vi "MeasureAndSaveData.vi"(0 "object in":refnum<class "AD2_SDK.lvclass">, 2 "tdms file":refnum<k34>, 5 "error in (no error)":errorcluster) -> (14 "object out":refnum<class "AD2_SDK.lvclass">, 17 "Channels array":waveform(dbl)[](array[waveform]), 19 "error out":errorcluster)   [LabVIEW 2023, in "AD2_SDK.lvclass"]
uses:
  AD2_SDK.lvclass
  AD2_SDK.lvclass/AD2_SDK.ctl
  <vilib>/measure/NI_MAPro.lvlib
  <vilib>/measure/matone.llb/Extract Single Tone Information 1 Chan.vi
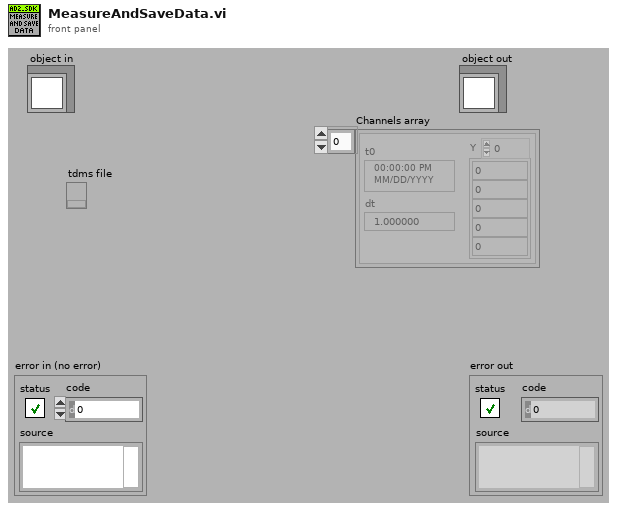
[diagram p1: front panel]
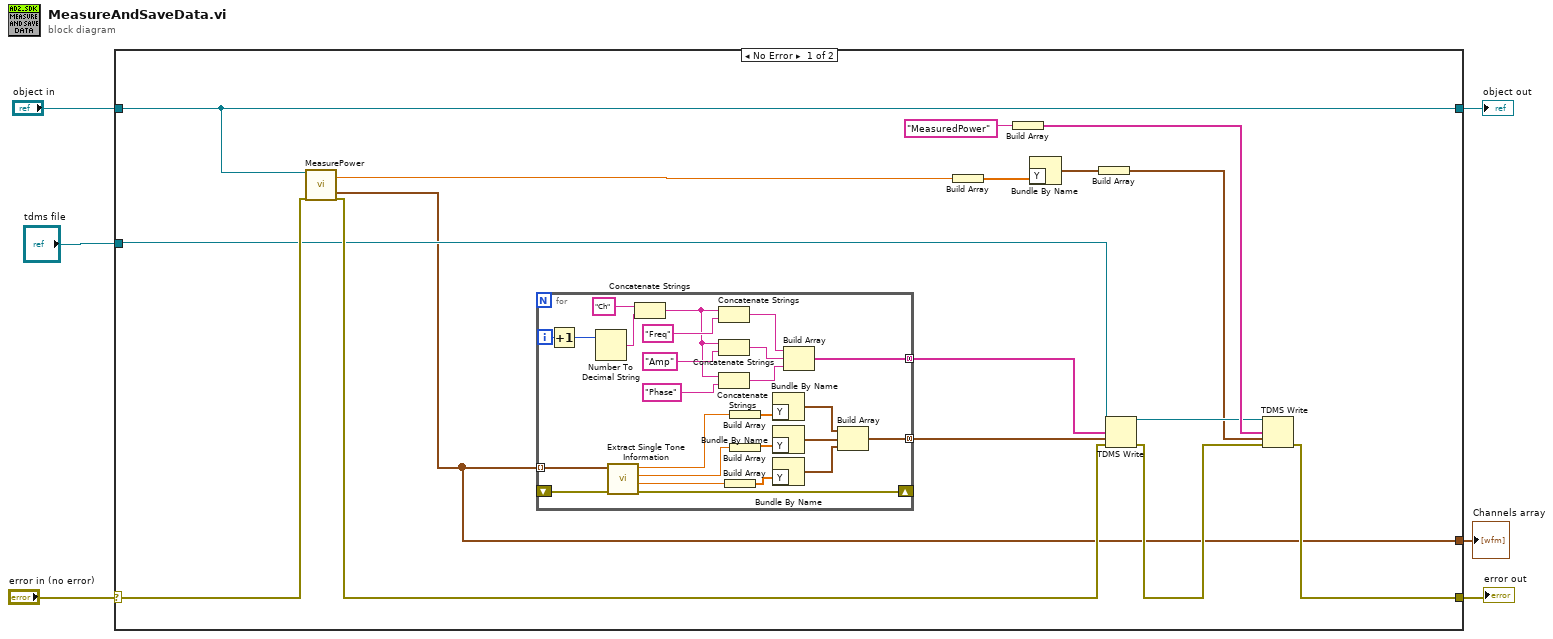
[diagram p0: block diagram]
diagram:
  n1 = case shown="No Error" "error in (no error)" {
    selector: "error in (no error)" -> [w21 w49]
    tunnel: [w11 w49] -> w5
    tunnel: [w22 w48] -> w3
    tunnel: "object in" -> [w22 w48]
    tunnel: "tdms file" -> [w9 _]
    tunnel: [w7 _] -> w1
    frame No Error {
      n2 = call-dynamic "MeasurePower.vi"("object in"=w22, "error in (no error)"=w21) -> ("Power (W)"=w16:dbl, "Channels array"=w7:waveform(dbl)[], "error out"=w18:errorcluster)  [unwired: 12 in, 3 out]
      n3 = for {
        tunnel: [w39] -> w20 mode=concatenating
        shift-right: [w34] -> _
        shift-left: _ -> [w35]
        tunnel: w7 -> [w33] mode=indexing
        tunnel: [w23] -> w19 mode=concatenating
        i -> [w45]
        n4 = Increment(x=w45) -> (x+1=w40:i32)
        n5 = Number To Decimal String(number=w40) -> (decimal integer string=w46:string)  [unwired: 1 in]
        n6 = call-poly <vilib>:"Extract Single Tone Information.vi"("error in (no error)"=w35, "time signal in"=w33) -> ("error out"=w34:errorcluster, "detected phase (deg)"=w28:dbl, "detected amplitude"=w29:dbl, "detected frequency"=w32:dbl)  [unwired: 4 in, 2 out]
        n7 = Concatenate Strings("Ch" ("string"), w46) -> (w38:string)
        n8 = Concatenate Strings(w38, "Freq") -> (w42:string)
        n9 = Concatenate Strings(w38, "Amp") -> (w41:string)
        n10 = Concatenate Strings(w38, "Phase") -> (w36:string)
        n11 = Build Array(w28) -> (w30:dbl[])
        n12 = Build Array(w32) -> (w31:dbl[])
        n13 = Build Array(w29) -> (w27:dbl[])
        n14 = Bundle By Name("Y"=w31) -> (w26:waveform(dbl))  [unwired: 1 in]
        n15 = Bundle By Name("Y"=w27) -> (w25:waveform(dbl))  [unwired: 1 in]
        n16 = Bundle By Name("Y"=w30) -> (w24:waveform(dbl))  [unwired: 1 in]
        n17 = Build Array(w42, w41, w36) -> (w39:string[])
        n18 = Build Array(w26, w25, w24) -> (w23:waveform(dbl)[])
      }
      n19 = Build Array(w16) -> (w17:dbl[])
      n20 = Build Array("MeasuredPower") -> (w14:string[])
      n21 = Bundle By Name("Y"=w17) -> (w13:waveform(dbl))  [unwired: 1 in]
      n22 = Build Array(w13) -> (w8:waveform(dbl)[])
      n23 = TDMS Write(0:w9, 7:w20, 9:w19, 11:w18) -> (4:w10:refnum<k34>, 15:w12:errorcluster)  [unwired: 2 in, 2 out]
      n24 = TDMS Write(0:w10, 7:w14, 9:w8, 11:w12) -> (15:w11:errorcluster)  [unwired: 2 in, 3 out]
    }
    frame Error {
    }
  }
  "error out" <- w5
  "object out" <- w3
  "Channels array" <- w1
